vi "Read IGObjectFactory.vi"(11 "Search in":refnum<class "Search.lvclass">) -> (2 "IGObjectFactory":refnum<class "IGObjectFactory.lvclass">, 3 "Search out":refnum<class "Search.lvclass">)   [LabVIEW 2016, in "Search.lvclass"]
uses:
  Search.lvclass
  IGObjectFactory/IGObjectFactory.lvclass
  Search.lvclass/Search.ctl
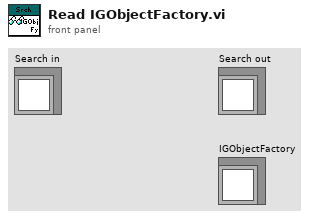
[diagram p1: front panel]
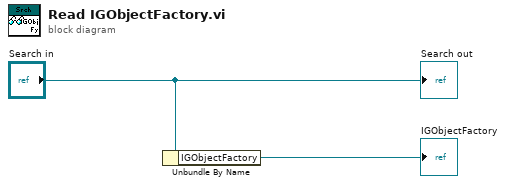
[diagram p0: block diagram]
diagram:
  n1 = Unbundle By Name("Search in") -> ("IGObjectFactory"=→"IGObjectFactory":refnum<class "IGObjectFactory.lvclass">)
  "Search out" <- "Search in"
